vi "niTuner Config Reference Clock.vi"(7 "error in":errorcluster, 9 "reference configuration":T1(ring)=enum."Internal", 10 "taskID in":i32 format="%.0x") -> (0 "error out":errorcluster, 3 "taskID out":i32 format="%.0x")   [LabVIEW 2011]
doc: "This VI configures the reference clock source. The PXI-5600 downconverter must lock to a timebase before entering the ready state."
uses:
  nipxi5600u.dll
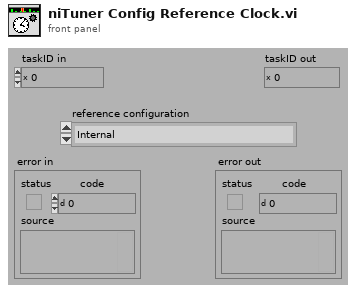
[diagram p1: front panel]
types:
  T1 = enum32{"Drive 10 MHz PXI Backplane Clock", "Internal", "Lock To 10 MHz PXI Backplane Clock", "External", "Drive 10 MHz PXI Backplane Clock External"}
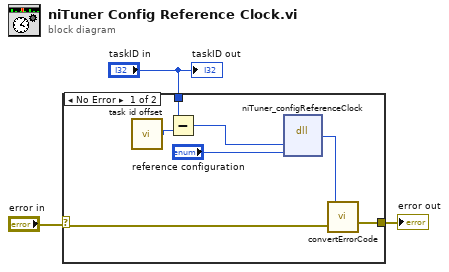
[diagram p0: block diagram]
diagram:
  n1 = case shown="No Error" "error in" {
    selector: "error in" -> [w9 w11]
    tunnel: [w8 w11] -> w2
    tunnel: "taskID in" -> [w6 _]
    frame No Error {
      n2 = call <instrlib>:"task id offset.vi"() -> ("taskID offset"=w7:i32)
      n3 = Subtract(x=w6, y=w7) -> (x-y=w5:i32)
      n4 = dll-call lib="nipxi5600u.dll" fn="niTuner_configReferenceClock"("taskID"=w5, "referenceConfiguration"="reference configuration") -> (w10:i32)  [unwired: 5 in, 2 out]
      n5 = call <instrlib>:"convertErrorCode.vi"("error in"=w9, "error code"=w10) -> ("error out"=w8:errorcluster)
    }
    frame Error {
    }
  }
  "error out" <- w2
  "taskID out" <- "taskID in"
